vi "delay judge.vi"(9 "Spec":dbl, 10 "Impedance Data":dbl[](array[numeric]), 11 "Time Array":dbl[](array[numeric])) -> (2 "result":bool, 3 "delay":dbl)   [LabVIEW 2011]
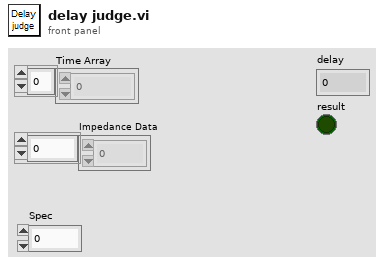
[diagram p1: front panel]
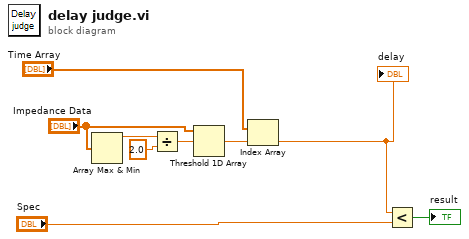
[diagram p0: block diagram]
diagram:
  n1 = Array Max & Min(array="Impedance Data") -> (max value=w6:dbl)  [unwired: 3 out]
  n2 = Divide(x=w6, y=2.0) -> (x/y=w4:dbl)
  n3 = Threshold 1D Array(2:w4, 3:"Impedance Data") -> (0:w7:dbl)  [unwired: 1 in]
  n4 = Index Array(array="Time Array", index=w7) -> (element=w3:dbl)
  "delay" <- w3
  n5 = Less?(x=w3, y="Spec") -> (x < y?=→"result":bool)
